vi "Logic_API_Hierarchy.vi"   [LabVIEW 2021]
uses:
  Support/AND/Bool/AND_Bool.lvclass
  Support/AND/I8/AND_I8.lvclass
  Support/AND/I16/AND_I16.lvclass
  Support/AND/I32/AND_I32.lvclass
  Support/AND/I64/AND_I64.lvclass
  Support/AND/U8/AND_U8.lvclass
  Support/AND/U16/AND_U16.lvclass
  Support/AND/U32/AND_U32.lvclass
  Support/AND/U64/AND_U64.lvclass
  Support/OR/Bool/OR_Bool.lvclass
  Support/NAND/Bool/NAND_Bool.lvclass
  Support/OR/I8/OR_I8.lvclass
  Support/OR/I16/OR_I16.lvclass
  Support/OR/I32/OR_I32.lvclass
  Support/OR/I64/OR_I64.lvclass
  Support/OR/U8/OR_U8.lvclass
  Support/OR/U16/OR_U16.lvclass
  Support/OR/U32/OR_U32.lvclass
  Support/OR/U64/OR_U64.lvclass
  Support/NAND/I8/NAND_I8.lvclass
  Support/EXOR/Bool/EXOR_Bool.lvclass
  Support/EXNOR/Bool/EXNOR_Bool.lvclass
  Support/NOR/Bool/NOR_Bool.lvclass
  Support/NAND/I16/NAND_I16.lvclass
  Support/NAND/I32/NAND_I32.lvclass
  Support/NAND/I64/NAND_I64.lvclass
  Support/NAND/U8/NAND_U8.lvclass
  Support/NAND/U16/NAND_U16.lvclass
  Support/NAND/U32/NAND_U32.lvclass
  Support/NAND/U64/NAND_U64.lvclass
  Support/NOR/I8/NOR_I8.lvclass
  Support/NOR/I16/NOR_I16.lvclass
  Support/NOR/I32/NOR_I32.lvclass
  Support/NOR/I64/NOR_I64.lvclass
  Support/NOR/U8/NOR_U8.lvclass
  Support/NOR/U16/NOR_U16.lvclass
  Support/NOR/U32/NOR_U32.lvclass
  Support/NOR/U64/NOR_U64.lvclass
  Support/NOT/Bool/NOT_Bool.lvclass
  Support/NOT/I8/NOT_I8.lvclass
  Support/NOT/I16/NOT_I16.lvclass
  Support/NOT/I32/NOT_I32.lvclass
  Support/NOT/I64/NOT_I64.lvclass
  Support/NOT/U8/NOT_U8.lvclass
  Support/NOT/U16/NOT_U16.lvclass
  Support/NOT/U32/NOT_U32.lvclass
  Support/NOT/U64/NOT_U64.lvclass
  Support/EXOR/I8/EXOR_I8.lvclass
  Support/EXOR/I16/EXOR_I16.lvclass
  Support/EXOR/I32/EXOR_I32.lvclass
  Support/EXOR/I64/EXOR_I64.lvclass
  Support/EXOR/U8/EXOR_U8.lvclass
  Support/EXOR/U16/EXOR_U16.lvclass
  Support/EXOR/U32/EXOR_U32.lvclass
  Support/EXOR/U64/EXOR_U64.lvclass
  Support/EXNOR/I8/EXNOR_I8.lvclass
  Support/EXNOR/I16/EXNOR_I16.lvclass
  Support/EXNOR/I32/EXNOR_I32.lvclass
  Support/EXNOR/I64/EXNOR_I64.lvclass
  Support/EXNOR/U8/EXNOR_U8.lvclass
  Support/EXNOR/U16/EXNOR_U16.lvclass
  Support/EXNOR/U32/EXNOR_U32.lvclass
  Support/EXNOR/U64/EXNOR_U64.lvclass
  Support/Function/Two Terminal/Boolean/AbsFunc_Two Term_Bool.lvclass
  Support/Function/Two Terminal/I8/AbsFunc_Two Term_I8.lvclass
  Support/Function/Two Terminal/I16/AbsFunc_Two Term_I16.lvclass
  Support/Function/Two Terminal/I32/AbsFunc_Two Term_I32.lvclass
  Support/Function/Two Terminal/I64/AbsFunc_Two Term_I64.lvclass
  Support/Function/Two Terminal/U8/AbsFunc_Two Term_U8.lvclass
  Support/Function/Two Terminal/U16/AbsFunc_Two Term_U16.lvclass
  Support/Function/Two Terminal/U32/AbsFunc_Two Term_U32.lvclass
  Support/Function/Two Terminal/U64/AbsFunc_Two Term_U64.lvclass
  Support/Function/One Terminal/Boolean/AbsFunc_One Term_Bool.lvclass
  Support/Function/One Terminal/I8/AbsFunc_One Term_I8.lvclass
  Support/Function/One Terminal/I16/AbsFunc_One Term_I16.lvclass
  Support/Function/One Terminal/I32/AbsFunc_One Term_I32.lvclass
  Support/Function/One Terminal/I64/AbsFunc_One Term_I64.lvclass
  Support/Function/One Terminal/U8/AbsFunc_One Term_U8.lvclass
  Support/Function/One Terminal/U16/AbsFunc_One Term_U16.lvclass
  Support/Function/One Terminal/U32/AbsFunc_One Term_U32.lvclass
  Support/Function/One Terminal/U64/AbsFunc_One Term_U64.lvclass
panel:
  # "SEE DIAGRAM\nFOR Hierarchy"
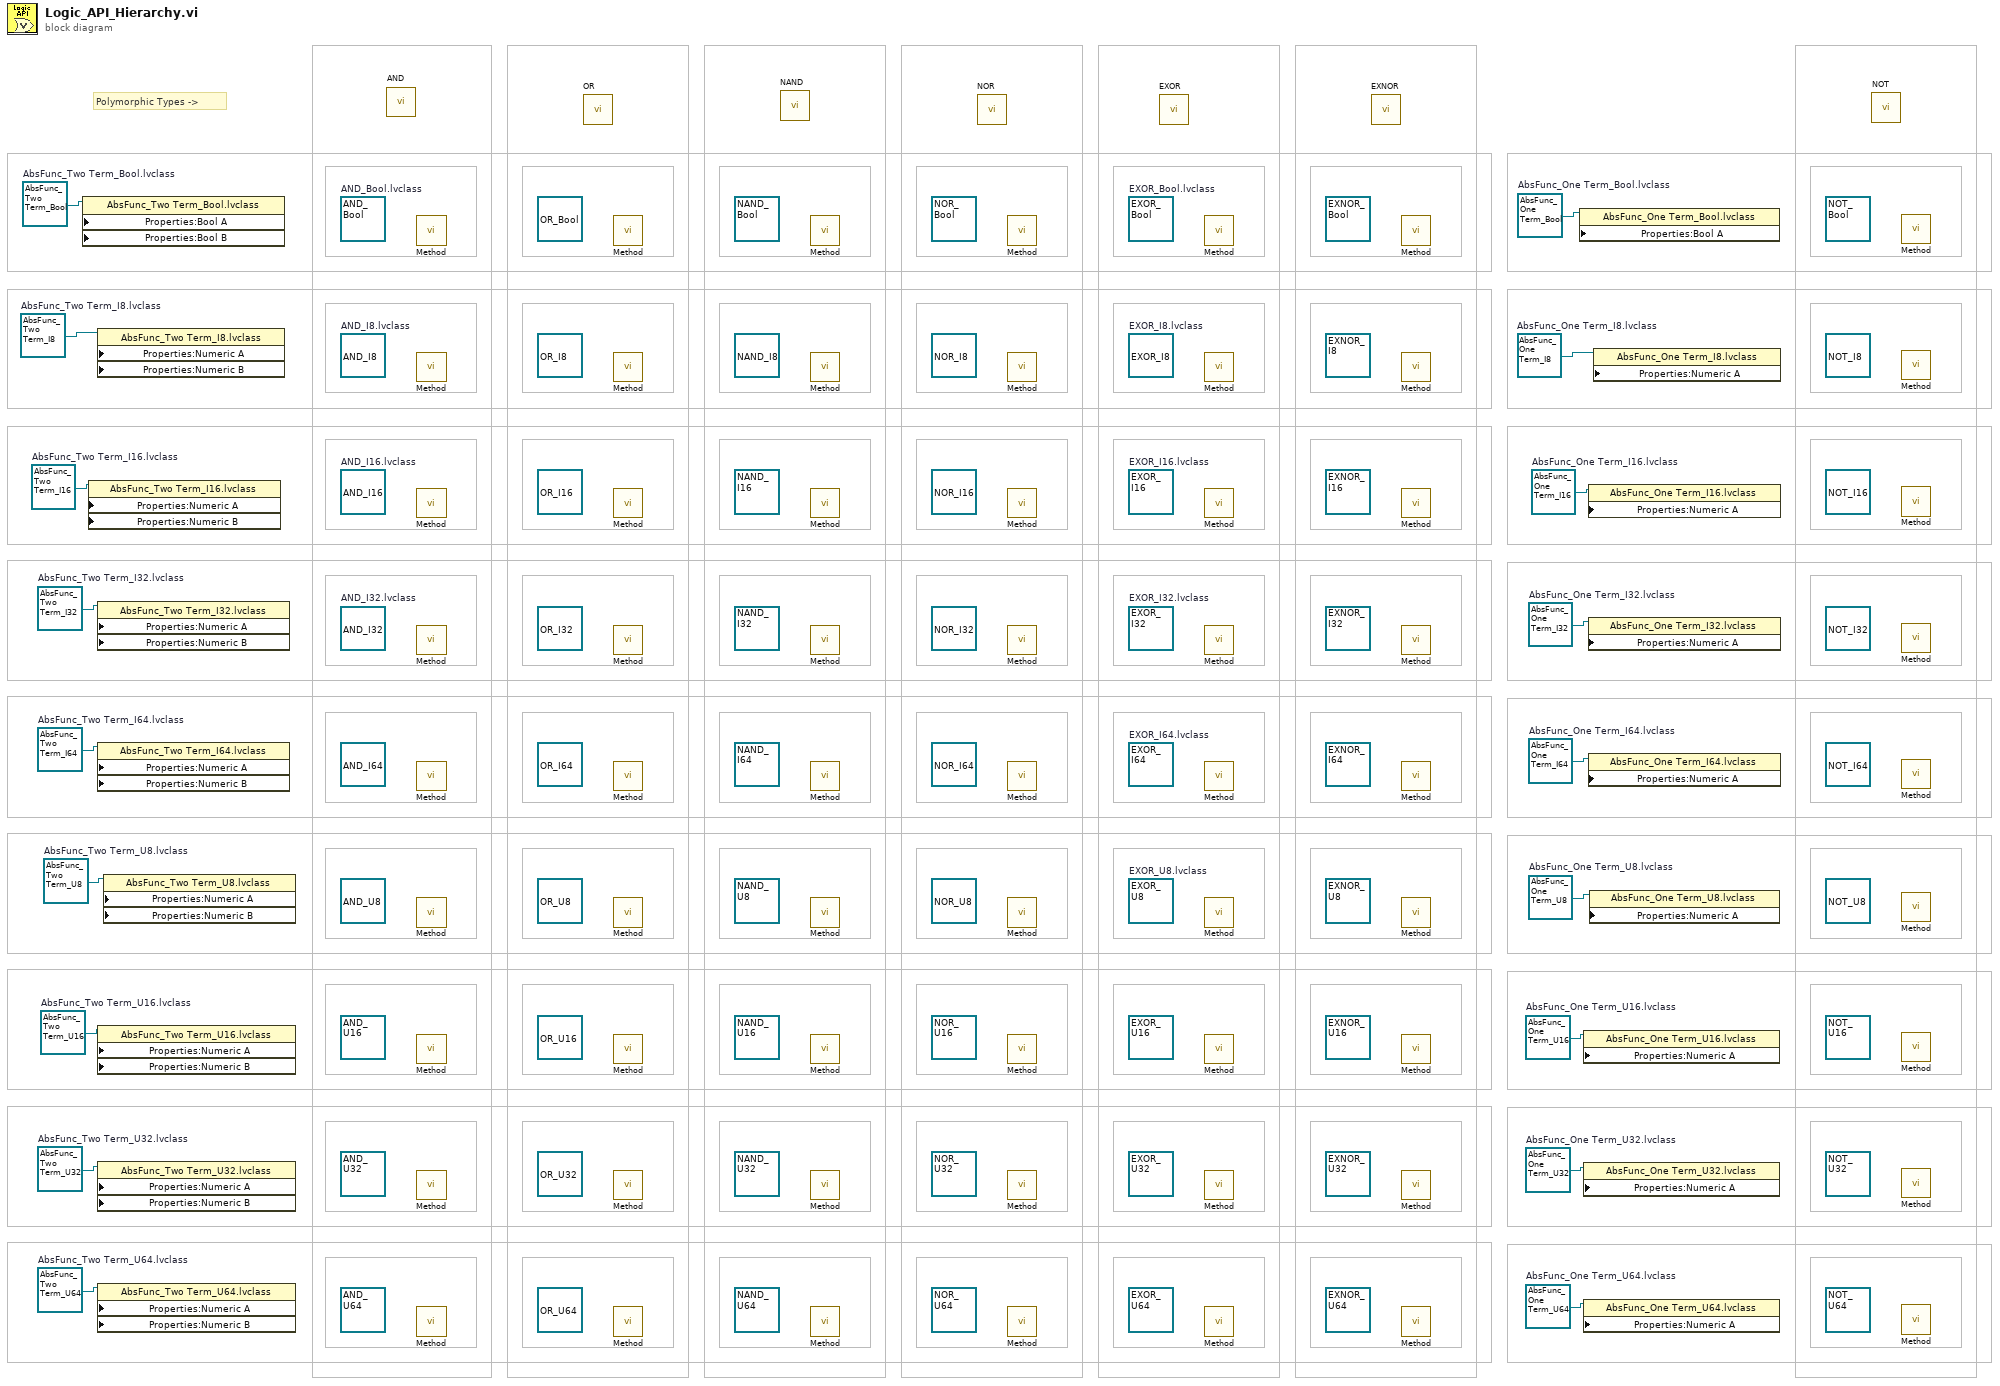
[diagram p0: block diagram]
diagram:
  w1 = refnum<class "AbsFunc_One Term_U64.lvclass"> refnum  # AbsFunc_One Term_U64.lvclass
  w2 = refnum<class "AbsFunc_One Term_U32.lvclass"> refnum  # AbsFunc_One Term_U32.lvclass
  w3 = refnum<class "AbsFunc_One Term_U16.lvclass"> refnum  # AbsFunc_One Term_U16.lvclass
  w4 = refnum<class "AbsFunc_One Term_U8.lvclass"> refnum  # AbsFunc_One Term_U8.lvclass
  w5 = refnum<class "AbsFunc_One Term_I64.lvclass"> refnum  # AbsFunc_One Term_I64.lvclass
  w6 = refnum<class "AbsFunc_One Term_I32.lvclass"> refnum  # AbsFunc_One Term_I32.lvclass
  w7 = refnum<class "AbsFunc_One Term_I16.lvclass"> refnum  # AbsFunc_One Term_I16.lvclass
  w8 = refnum<class "AbsFunc_One Term_I8.lvclass"> refnum  # AbsFunc_One Term_I8.lvclass
  w9 = refnum<class "AbsFunc_One Term_Bool.lvclass"> refnum  # AbsFunc_One Term_Bool.lvclass
  w10 = refnum<class "AbsFunc_Two Term_U64.lvclass"> refnum  # AbsFunc_Two Term_U64.lvclass
  w11 = refnum<class "AbsFunc_Two Term_U32.lvclass"> refnum  # AbsFunc_Two Term_U32.lvclass
  w12 = refnum<class "AbsFunc_Two Term_U16.lvclass"> refnum  # AbsFunc_Two Term_U16.lvclass
  w13 = refnum<class "AbsFunc_Two Term_U8.lvclass"> refnum  # AbsFunc_Two Term_U8.lvclass
  w14 = refnum<class "AbsFunc_Two Term_I64.lvclass"> refnum  # AbsFunc_Two Term_I64.lvclass
  w15 = refnum<class "AbsFunc_Two Term_I32.lvclass"> refnum  # AbsFunc_Two Term_I32.lvclass
  w16 = refnum<class "AbsFunc_Two Term_I16.lvclass"> refnum  # AbsFunc_Two Term_I16.lvclass
  w17 = refnum<class "AbsFunc_Two Term_I8.lvclass"> refnum  # AbsFunc_Two Term_I8.lvclass
  w18 = refnum<class "AbsFunc_Two Term_Bool.lvclass"> refnum  # AbsFunc_Two Term_Bool.lvclass
  (unwired) refnum<class "EXNOR_U64.lvclass"> refnum ("EXNOR_U64.lvclass")
  (unwired) refnum<class "EXNOR_U32.lvclass"> refnum ("EXNOR_U32.lvclass")
  (unwired) refnum<class "EXNOR_U16.lvclass"> refnum ("EXNOR_U16.lvclass")
  (unwired) refnum<class "EXNOR_U8.lvclass"> refnum ("EXNOR_U8.lvclass")
  (unwired) refnum<class "EXNOR_I64.lvclass"> refnum ("EXNOR_I64.lvclass")
  (unwired) refnum<class "EXNOR_I32.lvclass"> refnum ("EXNOR_I32.lvclass")
  (unwired) refnum<class "EXNOR_I16.lvclass"> refnum ("EXNOR_I16.lvclass")
  (unwired) refnum<class "EXNOR_I8.lvclass"> refnum ("EXNOR_I8.lvclass")
  (unwired) refnum<class "EXNOR_Bool.lvclass"> refnum ("EXNOR_Bool.lvclass")
  (unwired) refnum<class "EXOR_U64.lvclass"> refnum ("EXOR_U64.lvclass")
  (unwired) refnum<class "EXOR_U32.lvclass"> refnum ("EXOR_U32.lvclass")
  (unwired) refnum<class "EXOR_U16.lvclass"> refnum ("EXOR_U16.lvclass")
  (unwired) refnum<class "EXOR_U8.lvclass"> refnum  # EXOR_U8.lvclass
  (unwired) refnum<class "EXOR_I64.lvclass"> refnum  # EXOR_I64.lvclass
  (unwired) refnum<class "EXOR_I32.lvclass"> refnum  # EXOR_I32.lvclass
  (unwired) refnum<class "EXOR_I16.lvclass"> refnum  # EXOR_I16.lvclass
  (unwired) refnum<class "EXOR_I8.lvclass"> refnum  # EXOR_I8.lvclass
  (unwired) refnum<class "EXOR_Bool.lvclass"> refnum  # EXOR_Bool.lvclass
  (unwired) refnum<class "NOT_U64.lvclass"> refnum ("NOT_U64.lvclass")
  (unwired) refnum<class "NOT_U32.lvclass"> refnum ("NOT_U32.lvclass")
  (unwired) refnum<class "NOT_U16.lvclass"> refnum ("NOT_U16.lvclass")
  (unwired) refnum<class "NOT_U8.lvclass"> refnum ("NOT_U8.lvclass")
  (unwired) refnum<class "NOT_I64.lvclass"> refnum ("NOT_I64.lvclass")
  (unwired) refnum<class "NOT_I32.lvclass"> refnum ("NOT_I32.lvclass")
  (unwired) refnum<class "NOT_I16.lvclass"> refnum ("NOT_I16.lvclass")
  (unwired) refnum<class "NOT_I8.lvclass"> refnum ("NOT_I8.lvclass")
  (unwired) refnum<class "NOT_Bool.lvclass"> refnum ("NOT_Bool.lvclass")
  (unwired) refnum<class "NOR_U64.lvclass"> refnum ("NOR_U64.lvclass")
  (unwired) refnum<class "NOR_U32.lvclass"> refnum ("NOR_U32.lvclass")
  (unwired) refnum<class "NOR_U16.lvclass"> refnum ("NOR_U16.lvclass")
  (unwired) refnum<class "NOR_U8.lvclass"> refnum ("NOR_U8.lvclass")
  (unwired) refnum<class "NOR_I64.lvclass"> refnum ("NOR_I64.lvclass")
  (unwired) refnum<class "NOR_I32.lvclass"> refnum ("NOR_I32.lvclass")
  (unwired) refnum<class "NOR_I16.lvclass"> refnum ("NOR_I16.lvclass")
  (unwired) refnum<class "NOR_I8.lvclass"> refnum ("NOR_I8.lvclass")
  (unwired) refnum<class "NOR_Bool.lvclass"> refnum ("NOR_Bool.lvclass")
  (unwired) refnum<class "NAND_U64.lvclass"> refnum ("NAND_U64.lvclass")
  (unwired) refnum<class "NAND_U32.lvclass"> refnum ("NAND_U32.lvclass")
  (unwired) refnum<class "NAND_U16.lvclass"> refnum ("NAND_U16.lvclass")
  (unwired) refnum<class "NAND_U8.lvclass"> refnum ("NAND_U8.lvclass")
  (unwired) refnum<class "NAND_I64.lvclass"> refnum ("NAND_I64.lvclass")
  (unwired) refnum<class "NAND_I32.lvclass"> refnum ("NAND_I32.lvclass")
  (unwired) refnum<class "NAND_I16.lvclass"> refnum ("NAND_I16.lvclass")
  (unwired) refnum<class "NAND_I8.lvclass"> refnum ("NAND_I8.lvclass")
  (unwired) refnum<class "NAND_Bool.lvclass"> refnum ("NAND_Bool.lvclass")
  (unwired) refnum<class "OR_U64.lvclass"> refnum ("OR_U64.lvclass")
  (unwired) refnum<class "OR_U32.lvclass"> refnum ("OR_U32.lvclass")
  (unwired) refnum<class "OR_U16.lvclass"> refnum ("OR_U16.lvclass")
  (unwired) refnum<class "OR_U8.lvclass"> refnum ("OR_U8.lvclass")
  (unwired) refnum<class "OR_I64.lvclass"> refnum ("OR_I64.lvclass")
  (unwired) refnum<class "OR_I32.lvclass"> refnum ("OR_I32.lvclass")
  (unwired) refnum<class "OR_I16.lvclass"> refnum ("OR_I16.lvclass")
  (unwired) refnum<class "OR_I8.lvclass"> refnum ("OR_I8.lvclass")
  (unwired) refnum<class "OR_Bool.lvclass"> refnum ("OR_Bool.lvclass")
  (unwired) refnum<class "AND_U64.lvclass"> refnum ("AND_U64.lvclass")
  (unwired) refnum<class "AND_U32.lvclass"> refnum ("AND_U32.lvclass")
  (unwired) refnum<class "AND_U16.lvclass"> refnum ("AND_U16.lvclass")
  (unwired) refnum<class "AND_U8.lvclass"> refnum ("AND_U8.lvclass")
  (unwired) refnum<class "AND_I64.lvclass"> refnum ("AND_I64.lvclass")
  (unwired) refnum<class "AND_I32.lvclass"> refnum  # AND_I32.lvclass
  (unwired) refnum<class "AND_I16.lvclass"> refnum  # AND_I16.lvclass
  (unwired) refnum<class "AND_I8.lvclass"> refnum  # AND_I8.lvclass
  (unwired) refnum<class "AND_Bool.lvclass"> refnum  # AND_Bool.lvclass
  # "Polymorphic Types ->"
  n1 = property class="AbsFunc_Two Term_Bool.lvclass" props=["Properties:Bool A", "Properties:Bool B"](reference=w18) -> ()  [unwired: 3 in, 2 out]
  n2 = property class="AbsFunc_Two Term_I16.lvclass" props=["Properties:Numeric A", "Properties:Numeric B"](reference=w16) -> ()  [unwired: 3 in, 2 out]
  n3 = property class="AbsFunc_Two Term_I8.lvclass" props=["Properties:Numeric A", "Properties:Numeric B"](reference=w17) -> ()  [unwired: 3 in, 2 out]
  n4 = property class="AbsFunc_Two Term_I32.lvclass" props=["Properties:Numeric A", "Properties:Numeric B"](reference=w15) -> ()  [unwired: 3 in, 2 out]
  n5 = property class="AbsFunc_Two Term_I64.lvclass" props=["Properties:Numeric A", "Properties:Numeric B"](reference=w14) -> ()  [unwired: 3 in, 2 out]
  n6 = property class="AbsFunc_Two Term_U16.lvclass" props=["Properties:Numeric A", "Properties:Numeric B"](reference=w12) -> ()  [unwired: 3 in, 2 out]
  n7 = property class="AbsFunc_Two Term_U32.lvclass" props=["Properties:Numeric A", "Properties:Numeric B"](reference=w11) -> ()  [unwired: 3 in, 2 out]
  n8 = property class="AbsFunc_Two Term_U64.lvclass" props=["Properties:Numeric A", "Properties:Numeric B"](reference=w10) -> ()  [unwired: 3 in, 2 out]
  n9 = property class="AbsFunc_Two Term_U8.lvclass" props=["Properties:Numeric A", "Properties:Numeric B"](reference=w13) -> ()  [unwired: 3 in, 2 out]
  n10 = call-poly "AND.vi"() -> ()  [unwired: 6 in, 1 out]
  n11 = call "Method.vi"() -> ()  [unwired: 6 in, 1 out]
  n12 = call "Method.vi"() -> ()  [unwired: 6 in, 1 out]
  n13 = call "Method.vi"() -> ()  [unwired: 6 in, 1 out]
  n14 = call "Method.vi"() -> ()  [unwired: 6 in, 1 out]
  n15 = call "Method.vi"() -> ()  [unwired: 6 in, 1 out]
  n16 = call "Method.vi"() -> ()  [unwired: 6 in, 1 out]
  n17 = call "Method.vi"() -> ()  [unwired: 6 in, 1 out]
  n18 = call "Method.vi"() -> ()  [unwired: 6 in, 1 out]
  n19 = call "Method.vi"() -> ()  [unwired: 6 in, 1 out]
  n20 = call-poly "OR.vi"() -> ()  [unwired: 6 in, 1 out]
  n21 = call "Method.vi"() -> ()  [unwired: 6 in, 1 out]
  n22 = call "Method.vi"() -> ()  [unwired: 6 in, 1 out]
  n23 = call "Method.vi"() -> ()  [unwired: 6 in, 1 out]
  n24 = call "Method.vi"() -> ()  [unwired: 6 in, 1 out]
  n25 = call "Method.vi"() -> ()  [unwired: 6 in, 1 out]
  n26 = call "Method.vi"() -> ()  [unwired: 6 in, 1 out]
  n27 = call "Method.vi"() -> ()  [unwired: 6 in, 1 out]
  n28 = call "Method.vi"() -> ()  [unwired: 6 in, 1 out]
  n29 = call "Method.vi"() -> ()  [unwired: 6 in, 1 out]
  n30 = call-poly "NAND.vi"() -> ()  [unwired: 6 in, 1 out]
  n31 = call "Method.vi"() -> ()  [unwired: 6 in, 1 out]
  n32 = call "Method.vi"() -> ()  [unwired: 6 in, 1 out]
  n33 = call "Method.vi"() -> ()  [unwired: 6 in, 1 out]
  n34 = call "Method.vi"() -> ()  [unwired: 6 in, 1 out]
  n35 = call "Method.vi"() -> ()  [unwired: 6 in, 1 out]
  n36 = call "Method.vi"() -> ()  [unwired: 6 in, 1 out]
  n37 = call "Method.vi"() -> ()  [unwired: 6 in, 1 out]
  n38 = call "Method.vi"() -> ()  [unwired: 6 in, 1 out]
  n39 = call "Method.vi"() -> ()  [unwired: 6 in, 1 out]
  n40 = call-poly "NOR.vi"() -> ()  [unwired: 6 in, 1 out]
  n41 = call "Method.vi"() -> ()  [unwired: 6 in, 1 out]
  n42 = call "Method.vi"() -> ()  [unwired: 6 in, 1 out]
  n43 = call "Method.vi"() -> ()  [unwired: 6 in, 1 out]
  n44 = call "Method.vi"() -> ()  [unwired: 6 in, 1 out]
  n45 = call "Method.vi"() -> ()  [unwired: 6 in, 1 out]
  n46 = call "Method.vi"() -> ()  [unwired: 6 in, 1 out]
  n47 = call "Method.vi"() -> ()  [unwired: 6 in, 1 out]
  n48 = call "Method.vi"() -> ()  [unwired: 6 in, 1 out]
  n49 = call "Method.vi"() -> ()  [unwired: 6 in, 1 out]
  n50 = call-poly "EXOR.vi"() -> ()  [unwired: 6 in, 1 out]
  n51 = call "Method.vi"() -> ()  [unwired: 6 in, 1 out]
  n52 = call "Method.vi"() -> ()  [unwired: 6 in, 1 out]
  n53 = call "Method.vi"() -> ()  [unwired: 6 in, 1 out]
  n54 = call "Method.vi"() -> ()  [unwired: 6 in, 1 out]
  n55 = call "Method.vi"() -> ()  [unwired: 6 in, 1 out]
  n56 = call "Method.vi"() -> ()  [unwired: 6 in, 1 out]
  n57 = call "Method.vi"() -> ()  [unwired: 6 in, 1 out]
  n58 = call "Method.vi"() -> ()  [unwired: 6 in, 1 out]
  n59 = call "Method.vi"() -> ()  [unwired: 6 in, 1 out]
  n60 = call-poly "EXNOR.vi"() -> ()  [unwired: 6 in, 1 out]
  n61 = call "Method.vi"() -> ()  [unwired: 6 in, 1 out]
  n62 = call "Method.vi"() -> ()  [unwired: 6 in, 1 out]
  n63 = call "Method.vi"() -> ()  [unwired: 6 in, 1 out]
  n64 = call "Method.vi"() -> ()  [unwired: 6 in, 1 out]
  n65 = call "Method.vi"() -> ()  [unwired: 6 in, 1 out]
  n66 = call "Method.vi"() -> ()  [unwired: 6 in, 1 out]
  n67 = call "Method.vi"() -> ()  [unwired: 6 in, 1 out]
  n68 = call "Method.vi"() -> ()  [unwired: 6 in, 1 out]
  n69 = call "Method.vi"() -> ()  [unwired: 6 in, 1 out]
  n70 = property class="AbsFunc_One Term_Bool.lvclass" props=["Properties:Bool A"](reference=w9) -> ()  [unwired: 2 in, 2 out]
  n71 = property class="AbsFunc_One Term_U16.lvclass" props=["Properties:Numeric A"](reference=w3) -> ()  [unwired: 2 in, 2 out]
  n72 = property class="AbsFunc_One Term_U32.lvclass" props=["Properties:Numeric A"](reference=w2) -> ()  [unwired: 2 in, 2 out]
  n73 = property class="AbsFunc_One Term_U64.lvclass" props=["Properties:Numeric A"](reference=w1) -> ()  [unwired: 2 in, 2 out]
  n74 = property class="AbsFunc_One Term_I16.lvclass" props=["Properties:Numeric A"](reference=w7) -> ()  [unwired: 2 in, 2 out]
  n75 = property class="AbsFunc_One Term_I32.lvclass" props=["Properties:Numeric A"](reference=w6) -> ()  [unwired: 2 in, 2 out]
  n76 = property class="AbsFunc_One Term_I64.lvclass" props=["Properties:Numeric A"](reference=w5) -> ()  [unwired: 2 in, 2 out]
  n77 = property class="AbsFunc_One Term_U8.lvclass" props=["Properties:Numeric A"](reference=w4) -> ()  [unwired: 2 in, 2 out]
  n78 = property class="AbsFunc_One Term_I8.lvclass" props=["Properties:Numeric A"](reference=w8) -> ()  [unwired: 2 in, 2 out]
  n79 = call-poly "NOT.vi"() -> ()  [unwired: 5 in, 1 out]
  n80 = call "Method.vi"() -> ()  [unwired: 5 in, 1 out]
  n81 = call "Method.vi"() -> ()  [unwired: 5 in, 1 out]
  n82 = call "Method.vi"() -> ()  [unwired: 5 in, 1 out]
  n83 = call "Method.vi"() -> ()  [unwired: 5 in, 1 out]
  n84 = call "Method.vi"() -> ()  [unwired: 5 in, 1 out]
  n85 = call "Method.vi"() -> ()  [unwired: 5 in, 1 out]
  n86 = call "Method.vi"() -> ()  [unwired: 5 in, 1 out]
  n87 = call "Method.vi"() -> ()  [unwired: 5 in, 1 out]
  n88 = call "Method.vi"() -> ()  [unwired: 5 in, 1 out]
